vi "Execute Tests.vi"(6 "% complete":refnum<user-event>, 11 "Library in":refnum<vi>) -> (1 "Tests":string[](array[string]), 2 "execution times (ms)":u32[](array[numeric]), 3 "results":errorcluster[](array[cluster]))   [LabVIEW 2014, in "SQLite3LV Tests.lvlib"]
uses:
  SQLite3LV Tests.lvlib
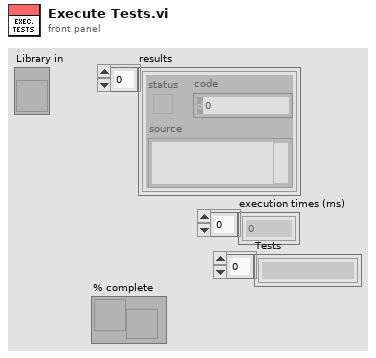
[diagram p1: front panel]
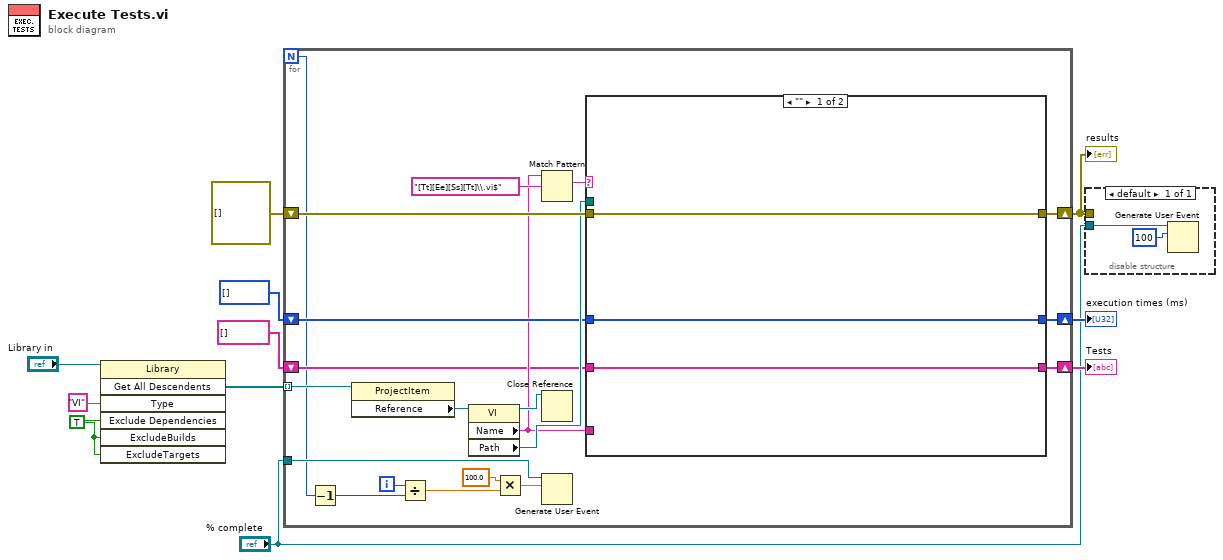
[diagram p0: block diagram]
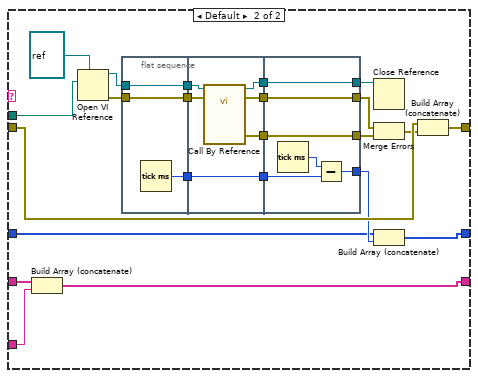
[diagram p2: hidden frame]
diagram:
  w9 = TRUE ("ExcludeDependencies")
  n1 = invoke class="Library" method="Get All Descendents"(reference="Library in", "Type"="VI", "Exclude Dependencies"=w9, "ExcludeBuilds"=w9, "ExcludeTargets"=w9) -> ("All Descendents"=w10:refnum<vi>[])  [unwired: 2 in, 6 out]
  n2 = for {
    N -> [w17]
    tunnel: w10 -> [w31] mode=indexing
    shift-right: [w27] -> w1
    shift-left: errorcluster[] [] -> [w26]
    shift-right: [w23] -> w6
    shift-left: u32[] [] -> [w22]
    shift-right: [w20] -> w3
    shift-left: string[] [] -> [w19]
    tunnel: "% complete" -> [w18]
    i -> [w16]
    n3 = Decrement(x=w17) -> (x-1=w15:i32)
    n4 = property class="ProjectItem"(reference=w31) -> ("Reference"=w30:refnum<vi>)  [unwired: 1 in, 2 out]
    n5 = Divide(x=w16, y=w15) -> (x/y=w14:dbl)
    n6 = property class="VI"(reference=w30) -> (reference out=w24:refnum<vi>, "Name"=w21:string, "Path"=w25:path)  [unwired: 1 in, 1 out]
    n7 = Multiply(x=100.0, y=w14) -> (x*y=w12:dbl)
    n8 = Match Pattern(string=w21, regular expression="[Tt][Ee][Ss][Tt]\\.vi$") -> (match substring=w28:string)  [unwired: 1 in, 3 out]
    n9 = Close Reference(reference=w24) -> ()  [unwired: 1 in, 1 out]
    n10 = Generate User Event(user event=w18, event data cluster=w12) -> ()  [unwired: 2 in, 2 out]
    n11 = case shown="\"\"" w28 {
      tunnel: [w34 w57] -> w27
      tunnel: w26 -> [w34 w56]
      tunnel: w25 -> [_ w54]
      tunnel: [w33 w39] -> w23
      tunnel: w22 -> [w33 w38]
      tunnel: w21 -> [_ w37]
      tunnel: [w32 w36] -> w20
      tunnel: w19 -> [w32 w35]
      frame "" {
      }
      frame Default {
        n12 = Build Array (concatenate)(w35, w37) -> (w36:string[])
        n13 = Open VI Reference(type specifier VI Refnum (for type only)=refnum<vi> refnum, vi path=w54) -> (vi reference=w50:refnum<vi>, error out=w53:errorcluster)  [unwired: 4 in]
        n14 = flat-sequence {
          tunnel: w50 -> [w59]
          tunnel: w53 -> [w60]
          tunnel: [w60] -> w44
          tunnel: [w59] -> w43
          tunnel: [w58] -> w41
          tunnel: [w65] -> w47
          tunnel: [w64] -> w46
          tunnel: [w62] -> w45
          tunnel: w44 -> [w66]
          tunnel: w43 -> [w63]
          tunnel: [w61] -> w42
          tunnel: w41 -> [w61]
          tunnel: [w70] -> w48
          tunnel: [w71] -> w51
          tunnel: [w72] -> w52
          tunnel: w47 -> [w72]
          tunnel: w46 -> [w71]
          tunnel: w45 -> [w70]
          tunnel: w42 -> [w68]
          tunnel: [w67] -> w40
          frame #0 {
            n15 = Tick Count (ms)() -> (millisecond timer value=w58:u32)
          }
          frame #1 {
            n16 = call-by-ref "?"(reference=w63, error in=w66) -> (reference out=w62:refnum<vi>, error out=w65:errorcluster, 0:"error out"=w64:errorcluster)  [unwired: 11 in]
          }
          frame #2 {
            n17 = Tick Count (ms)() -> (millisecond timer value=w69:u32)
            n18 = Subtract(x=w69, y=w68) -> (x-y=w67:u32)
          }
        }
        n19 = Close Reference(reference=w48) -> ()  [unwired: 1 in, 1 out]
        n20 = Merge Errors(w52, w51) -> (w49:errorcluster)
        n21 = Build Array (concatenate)(w38, w40) -> (w39:u32[])
        n22 = Build Array (concatenate)(w56, w49) -> (w57:errorcluster[])
      }
    }
  }
  "results" <- w1
  "execution times (ms)" <- w6
  "Tests" <- w3
  n23 = disable-structure shown="default" {
    disable-tunnel: "% complete" -> [w74]
    disable-tunnel: w1 -> [_]
    frame Enabled {
      n24 = Generate User Event(user event=w74, event data cluster=100 ("x")) -> ()  [unwired: 2 in, 2 out]
    }
  }
